vi "AH_READ.VI"(0 "AH2500A address":string="20") -> (1 "capacitance":dbl=nan format="%.8f", 2 "loss":dbl=nan format="%.8f")   [LabVIEW 2018]
panel:
  out "Vexc":dbl=nan format="%.8f"
  out "out string":string
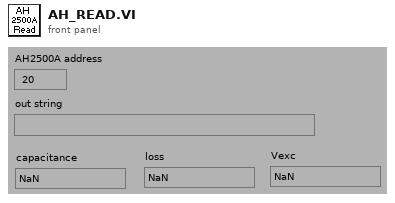
[diagram p1: front panel]
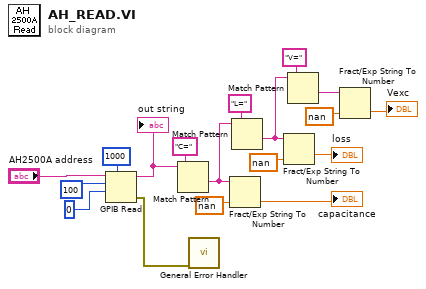
[diagram p0: block diagram]
diagram:
  n1 = GPIB Read(0:"AH2500A address", 1:100, 2:i16 0, 4:1000 ("timeout ms (488.2 global)")) -> (5:w13:string, 7:w1:errorcluster)  [unwired: 1 in, 1 out]
  "out string" <- w13
  n2 = Match Pattern(string=w13, regular expression="C=") -> (after substring=w8:string)  [unwired: 1 in, 3 out]
  n3 = call <vilib>:"General Error Handler.vi"("error in (no error)"=w1) -> ()  [unwired: 10 in, 5 out]
  n4 = Fract/Exp String To Number(string=w8, default (0 dbl)=nan) -> (number=→"capacitance":dbl)  [unwired: 2 in, 1 out]
  n5 = Match Pattern(string=w8, regular expression="L=") -> (after substring=w3:string)  [unwired: 1 in, 3 out]
  n6 = Fract/Exp String To Number(string=w3, default (0 dbl)=nan) -> (number=→"loss":dbl)  [unwired: 2 in, 1 out]
  n7 = Match Pattern(string=w3, regular expression="V=") -> (after substring=w6:string)  [unwired: 1 in, 3 out]
  n8 = Fract/Exp String To Number(string=w6, default (0 dbl)=nan) -> (number=→"Vexc":dbl)  [unwired: 2 in, 1 out]
